vi "poup_up_erro_login.vi"() -> ()   [LabVIEW 2016]
panel:
  in  "OK":bool
  # "usuário já cadastrado"
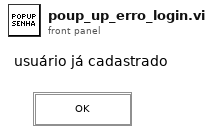
[diagram p1: front panel]
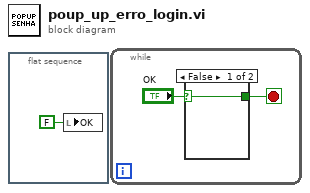
[diagram p0: block diagram]
diagram:
  n1 = flat-sequence {
    frame #0 {
      n2 = local write "OK"(FALSE ("OK")) -> ()
    }
  }
  n3 = while {
    stop <- w2 stop-if-true
    n4 = case shown="False" "OK" {
      selector: "OK" -> [w4 w5]
      tunnel: [w4 w5] -> w2
      frame False {
      }
      frame True {
      }
    }
  }
